vi "Construct.vi"(8 "error in (no error)":errorcluster, 9 "Menu Path (Relative)":path, 10 "Resource Data ref":refnum<data-value>, 11 "LVProject File Path":path) -> (0 "error out":errorcluster, 3 "Menu Data out":refnum<class "Menu Data.lvclass">)   [LabVIEW 2013, in "SET Project Data.lvlib" / "Menu Data.lvclass"]
uses:
  Menu Data.lvclass
  Resource Data Class/Resource Data.lvclass
  Menu Data.lvclass/Menu Data.ctl
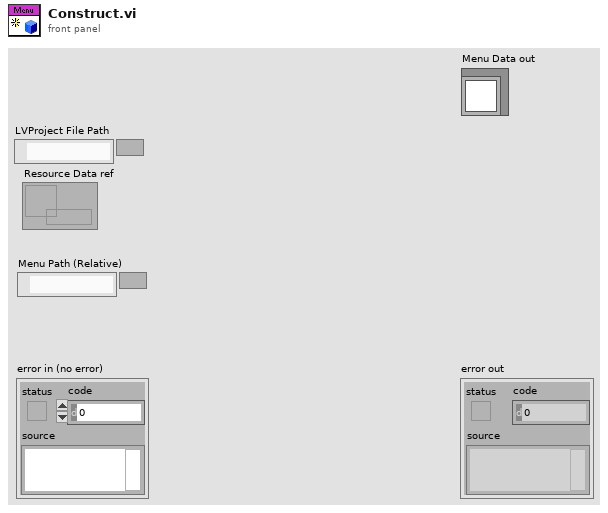
[diagram p1: front panel]
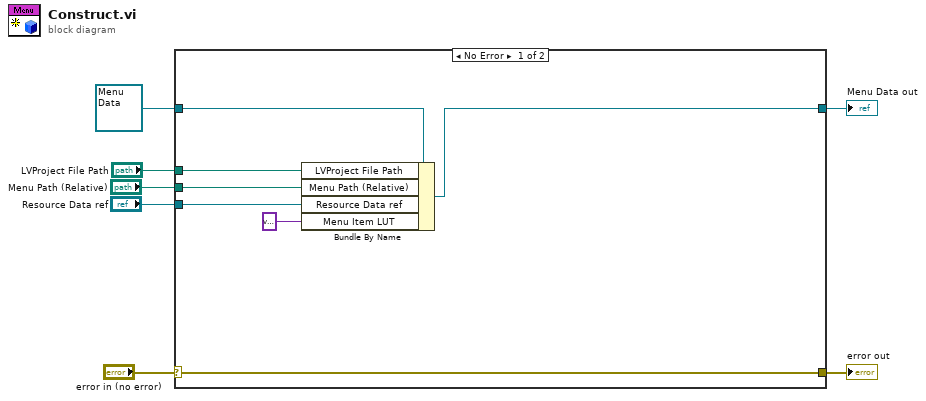
[diagram p0: block diagram]
diagram:
  n1 = case shown="No Error" "error in (no error)" {
    selector: "error in (no error)" -> [w14 w16]
    tunnel: [w14 w16] -> w6
    tunnel: [w12 w15] -> w4
    tunnel: refnum<class "Menu Data.lvclass"> refnum ("Menu Data in") -> [w13 w15]
    tunnel: "Menu Path (Relative)" -> [w11 _]
    tunnel: "Resource Data ref" -> [w10 _]
    tunnel: "LVProject File Path" -> [w8 _]
    frame No Error {
      n2 = Bundle By Name(cluster=w13, "LVProject File Path"=w8, "Menu Path (Relative)"=w11, "Resource Data ref"=w10, "Menu Item LUT"=variant ("GObject LUT")) -> (w12:refnum<class "Menu Data.lvclass">)
    }
    frame Error {
    }
  }
  "error out" <- w6
  "Menu Data out" <- w4
